vi "SetSRCreationDateStart(SubVI).vi"(10 "Date":timestamp, 11 "HTTP string":string) -> (3 "result string":string)   [LabVIEW 2017, in "MainFrameLib.lvlib"]
uses:
  MainFrameLib.lvlib
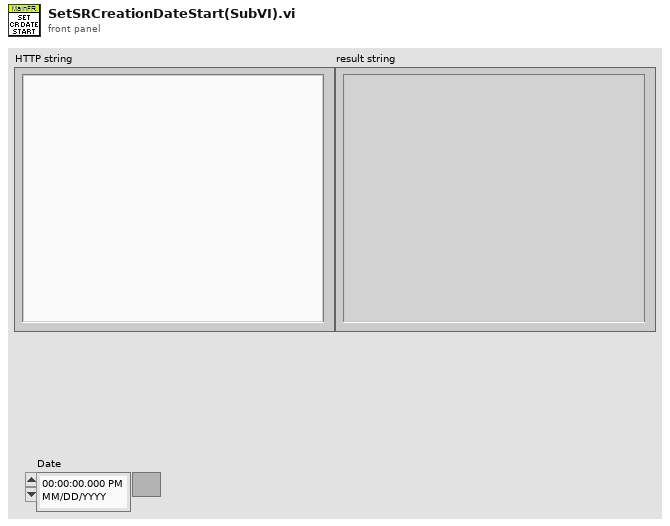
[diagram p1: front panel]
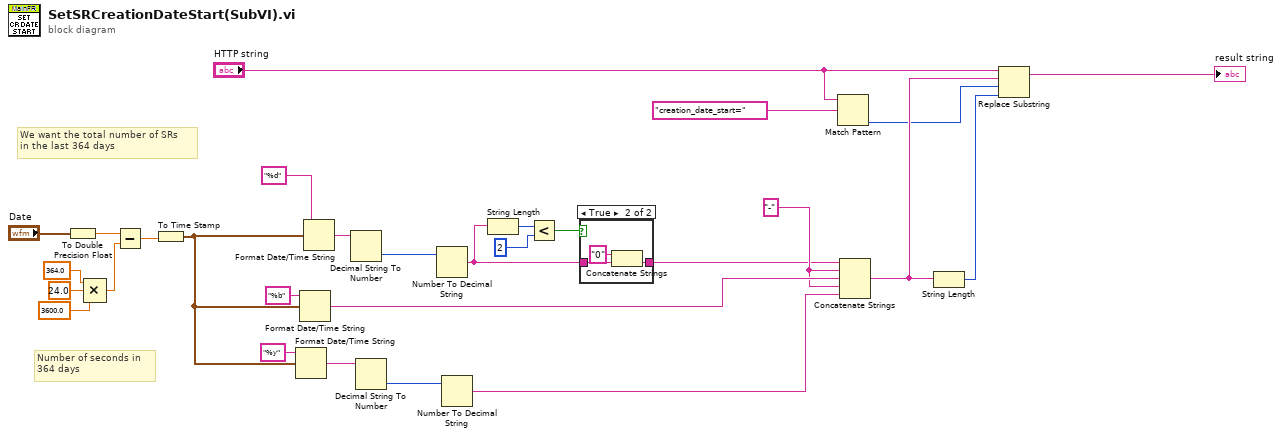
[diagram p0: block diagram]
diagram:
  w21 = "-" ("string")
  # "We want the total number of SRs \nin the last 364 days"
  # "Number of seconds in\n364 days"
  n1 = To Double Precision Float(number="Date") -> (double precision float=w8:dbl)
  n2 = Compound Arithmetic op=MULTIPLY(364.0 ("value"), 24.0 ("value"), 3600.0 ("value")) -> (w7:dbl)
  n3 = Subtract(x=w8, y=w7) -> (x-y=w3:dbl)
  n4 = To Time Stamp(1:w3) -> (0:w2:timestamp)
  n5 = Format Date/Time String(time format string (%c)="%y", seconds (now)=w2) -> (date/time string=w25:string)  [unwired: 1 in]
  n6 = Format Date/Time String(time format string (%c)="%b", seconds (now)=w2) -> (date/time string=w27:string)  [unwired: 1 in]
  n7 = Format Date/Time String(time format string (%c)="%d", seconds (now)=w2) -> (date/time string=w16:string)  [unwired: 1 in]
  n8 = Decimal String To Number(string=w16) -> (number=w10:i32)  [unwired: 2 in, 1 out]
  n9 = Decimal String To Number(string=w25) -> (number=w1:i32)  [unwired: 2 in, 1 out]
  n10 = Number To Decimal String(number=w10) -> (decimal integer string=w12:string)  [unwired: 1 in]
  n11 = Number To Decimal String(number=w1) -> (decimal integer string=w26:string)  [unwired: 1 in]
  n12 = String Length(string=w12) -> (length=w15:i32)
  n13 = Less?(x=w15, y=2) -> (x < y?=w13:bool)
  n14 = case shown="True" w13 {
    tunnel: w12 -> [w30 w33]
    tunnel: [w30 w31] -> w11
    frame False {
    }
    frame True {
      n15 = Concatenate Strings("0" ("string"), w33) -> (w31:string)
    }
  }
  n16 = Match Pattern(string="HTTP string", regular expression="creation_date_start=") -> (offset past match=w18:i32)  [unwired: 1 in, 3 out]
  n17 = Concatenate Strings(w11, w21, w27, w21, w26) -> (w28:string)
  n18 = String Length(string=w28) -> (length=w20:i32)
  n19 = Replace Substring(2:w20, 3:w18, 4:w28, 5:"HTTP string") -> (1:→"result string":string)  [unwired: 1 out]
